vi "CreateMethodNames.vi"(0 "_Method":i32[](array[numeric]), 2 "_Property":string[](array[string]), 3 "Item Names":string[](array[string]), 4 "Use Read/Write":bool) -> (5 "MethodNames":string[](array[string]), 6 "Attribute/PropertyNames":string[](array[string]))   [LabVIEW 2016, in "ClassWriterNative.lvclass"]
uses:
  <resource>/Framework/Providers/Open_GDS/ClassProviders/Provider_LvNativeClass/ClassWriterNative_class/ClassWriterNative.lvclass
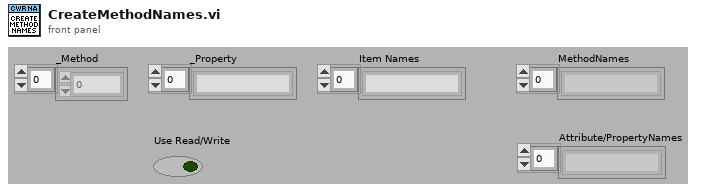
[diagram p1: front panel]
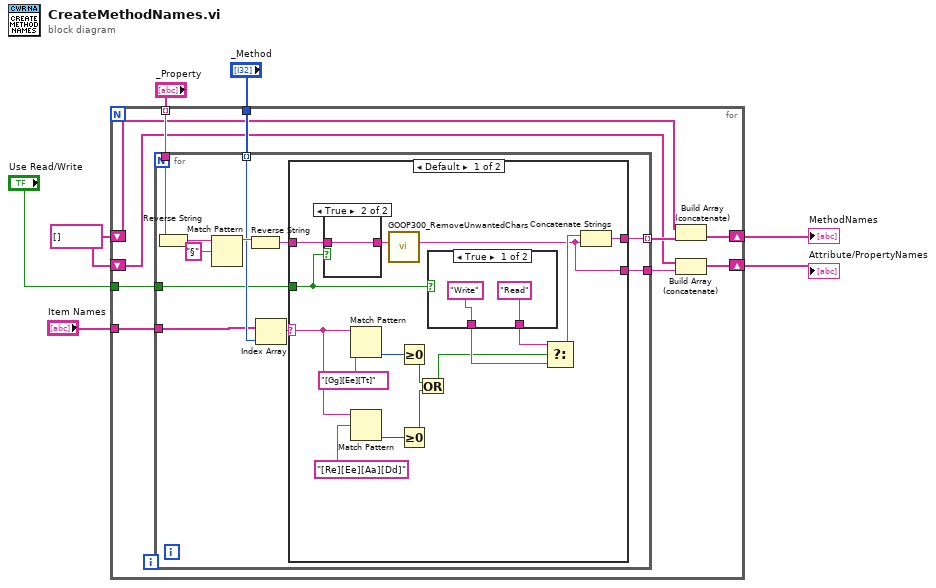
[diagram p0: block diagram]
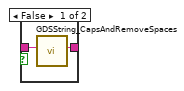
[diagram p2: hidden frame]
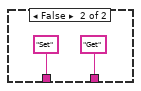
[diagram p3: hidden frame]
diagram:
  w2 = string[] []
  n1 = for {
    tunnel: "_Property" -> [w17] mode=indexing
    tunnel: "_Method" -> [w16]
    shift-right: [w14] -> w7
    shift-left: w2 -> [w13]
    tunnel: "Item Names" -> [w12]
    tunnel: "Use Read/Write" -> [w11]
    shift-right: [w10] -> w1
    shift-left: w2 -> [w8]
    n2 = for {
      tunnel: w17 -> [w28]
      tunnel: w16 -> [w22] mode=indexing
      tunnel: [w21] -> w15 mode=indexing
      tunnel: w12 -> [w20]
      tunnel: w11 -> [w19]
      tunnel: [w18] -> w9
      n3 = Reverse String(1:w28) -> (0:w27:string)
      n4 = Match Pattern(string=w27, regular expression="§") -> (before substring=w25:string)  [unwired: 1 in, 3 out]
      n5 = Reverse String(1:w25) -> (0:w23:string)
      n6 = Index Array(array=w20, index=w22) -> (element=w24:string)
      n7 = case shown="Default" w24 {
        selector: w24 -> [w35 _]
        tunnel: w23 -> [w39 _]
        tunnel: [w37 _] -> w21
        tunnel: w19 -> [w29 _]
        tunnel: [w30 _] -> w18
        frame Default {
          n8 = case shown="True" w29 {
            tunnel: w39 -> [w46 w47]
            tunnel: [w45 w47] -> w38
            frame False {
              n9 = call <resource>:"GDSString_CapsAndRemoveSpaces.vi"("String"=w46) -> ("concatenated string"=w45:string)  [unwired: 10 in]
            }
            frame True {
            }
          }
          n10 = Match Pattern(string=w35, regular expression="[Gg][Ee][Tt]") -> (offset past match=w43:i32)  [unwired: 1 in, 3 out]
          n11 = Match Pattern(string=w35, regular expression="[Re][Ee][Aa][Dd]") -> (offset past match=w34:i32)  [unwired: 1 in, 3 out]
          n12 = call <resource>:"GOOP300_RemoveUnwantedChars.vi"("StringIn"=w38) -> ("StringOut"=w30:string)  [unwired: 10 in]
          n13 = Greater Or Equal To 0?(x=w43) -> (x >= 0?=w32:bool)
          n14 = Greater Or Equal To 0?(x=w34) -> (x >= 0?=w33:bool)
          n15 = Or(x=w32, y=w33) -> (x .or. y?=w31:bool)
          n16 = case shown="True" w29 {
            tunnel: ["Read" ("regular expression") "Get" ("regular expression")] -> w42
            tunnel: ["Write" ("regular expression") "Set" ("regular expression")] -> w41
            frame True {
            }
            frame False {
            }
          }
          n17 = Select(t=w42, s=w31, f=w41) -> (s? t:f=w40:string)
          n18 = Concatenate Strings(w40, w30) -> (w37:string)
        }
        frame "" {
        }
      }
    }
    n19 = Build Array (concatenate)(w13, w15) -> (w14:string[])
    n20 = Build Array (concatenate)(w8, w9) -> (w10:string[])
  }
  "MethodNames" <- w7
  "Attribute/PropertyNames" <- w1
